vi "Untitled 3 (SubVI).vi"(8 "error in (no error)":errorcluster) -> (0 "error out":errorcluster, 2 "Array":u16[](array[numeric]), 3 "UP_Value":u16[](array[numeric]))   [LabVIEW 2016]
uses:
  <vilib>/myRIO/Instrument Drivers/Onboard IO/I2C/typedefs/I2C User Configuration.ctl
  <vilib>/myRIO/Instrument Drivers/Onboard IO/I2C/typedefs/I2C Transfer Rate.ctl
  <vilib>/myRIO/Instrument Drivers/Onboard IO/I2C/typedefs/I2C Reference.ctl
  <vilib>/myRIO/Common/Instrument Driver Framework/Utilities/typedefs/myRIO Generic Hardware Reference.ctl
  <vilib>/myRIO/Common/Instrument Driver Framework/Utilities/typedefs/Hardware Version Enum.ctl
  <vilib>/myRIO/Common/Instrument Driver Framework/Utilities/typedefs/myRIO v1.0 Reference.ctl
  <vilib>/myRIO/Common/Instrument Driver Framework/Utilities/typedefs/Generic FPGA Reference.ctl
  <vilib>/myRIO/Common/Instrument Driver Framework/myRIO v1.0/I2C/typedefs/I2C Channels Enum.ctl
  <vilib>/myRIO/Instrument Drivers/Onboard IO/I2C/typedefs/I2C Configuration.ctl
  <vilib>/userdefined/High Color/nirio_resource_hc.ctl
  <vilib>/myRIO/Common/Instrument Driver Framework/Utilities/vis/Is FPGA Ref Available.vi
  <vilib>/myRIO/Common/Instrument Driver Framework/myRIO v1.0/I2C/vis/myRIO v1.1 Open I2C.vi
  <vilib>/myRIO/Instrument Drivers/Onboard IO/I2C/vis/Configure.vi
  <vilib>/myRIO/Instrument Drivers/Onboard IO/I2C/vis/Write.vi
  <vilib>/myRIO/Instrument Drivers/Onboard IO/I2C/vis/Write Read.vi
  <vilib>/myRIO/Common/Instrument Driver Framework/Utilities/vis/Validate Channels.vi
  <vilib>/myRIO/Common/Instrument Driver Framework/myRIO v1.0/I2C/vis/myRIO v1.0 Reserve I2C.vi
  <vilib>/myRIO/Common/Instrument Driver Framework/myRIO v1.0/I2C/vis/myRIO v1.0 Build MUX Configuration I2C.vi
  <vilib>/myRIO/Common/Instrument Driver Framework/myRIO v1.0/Resource Manager/vis/myRIO v1.0 Reserve Channel List.vi
  <vilib>/myRIO/Common/Instrument Driver Framework/myRIO v1.0/Resource Manager/vis/myRIO v1.0 Create Configuration List.vi
  <vilib>/myRIO/Common/Instrument Driver Framework/myRIO v1.0/Resource Manager/vis/myRIO v1.0 Reserve Channel.vi
  <vilib>/myRIO/Common/Instrument Driver Framework/myRIO v1.0/Resource Manager/vis/myRIO v1.0 Unreserve Channel.vi
  <vilib>/myRIO/Common/Instrument Driver Framework/myRIO v1.0/Resource Manager/vis/myRIO v1.0 Build Mutex Name.vi
  <vilib>/Utility/VariantDataType/GetNumericInfo.vi
  <vilib>/Utility/error.llb/Error Cluster From Error Code.vi
  <vilib>/myRIO/Common/Instrument Driver Framework/myRIO v1.0/myRIO v1.1 Open.vi
  <vilib>/myRIO/Common/Instrument Driver Framework/Utilities/vis/IO Manager.vi
  <vilib>/myRIO/Common/Instrument Driver Framework/Utilities/vis/Configuration Manager.vi
  <vilib>/myRIO/Common/Instrument Driver Framework/myRIO v1.0/Resource Manager/vis/myRIO v1.0 Configure IO.vi
  <vilib>/myRIO/Common/Instrument Driver Framework/myRIO v1.0/myRIO v1.0 Close.vi
  <vilib>/myRIO/Common/Instrument Driver Framework/myRIO v1.0/I2C/vis/myRIO v1.0 Configure I2C.vi
  <vilib>/myRIO/Common/Instrument Driver Framework/myRIO v1.0/I2C/vis/myRIO v1.0 Write I2C.vi
  <vilib>/myRIO/Common/Instrument Driver Framework/myRIO v1.0/I2C/vis/myRIO v1.0 Read I2C.vi
  <vilib>/myRIO/Express VI/Onboard IO/I2C/I2C Express VI.xnode
  <vilib>/myRIO/Instrument Drivers/Onboard IO/I2C/vis/myRIO I2C Open.xnode
  <vilib>/myRIO/Instrument Drivers/Onboard IO/I2C/I2C.lvlib
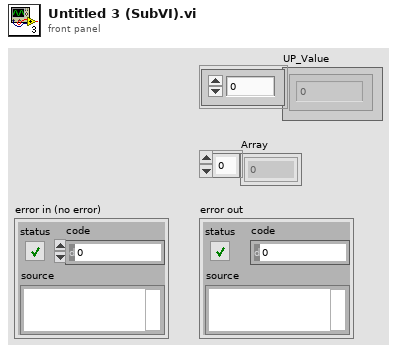
[diagram p1: front panel]
types:
  T1 = typedef "I2C.lvlib/I2C Reference.ctl" = cluster{"myRIO Reference":T2, "I2C Channels Enum":T6, "I2C Configuration":T7}
  T2 = typedef "myRIO Generic Hardware Reference.ctl" = cluster{"myRIO Model":T3, "myRIO Hardware Reference":T4}
  T3 = typedef "Hardware Version Enum.ctl" = enum16{"Unknown", "myRIO-1900", "myRIO-1950", "roboRIO", "NI ELVIS RIO CM"}
  T4 = typedef "myRIO v1.0 Reference.ctl" = cluster{"Generic FPGA Reference":T5, "Allow multiple opens":bool}
  T5 = typedef "Generic FPGA Reference.ctl" = refnum<k20>
  T6 = typedef "I2C Channels Enum.ctl" = enum16{"Not Connected", "A/I2C", "B/I2C", "I2C/I2C"}
  T7 = typedef "I2C.lvlib/I2C Configuration.ctl" = cluster{"I2C Transfer Rate":T8}
  T8 = typedef "I2C.lvlib/I2C Transfer Rate.ctl" = enum16{"Standard mode (100 kbps)", "Fast mode (400 kbps)"}
  T9 = typedef "I2C.lvlib/I2C User Configuration.ctl" = cluster{"I2C Transfer Rate":T8}
  T10 = typedef "nirio_resource_hc.ctl" = tag
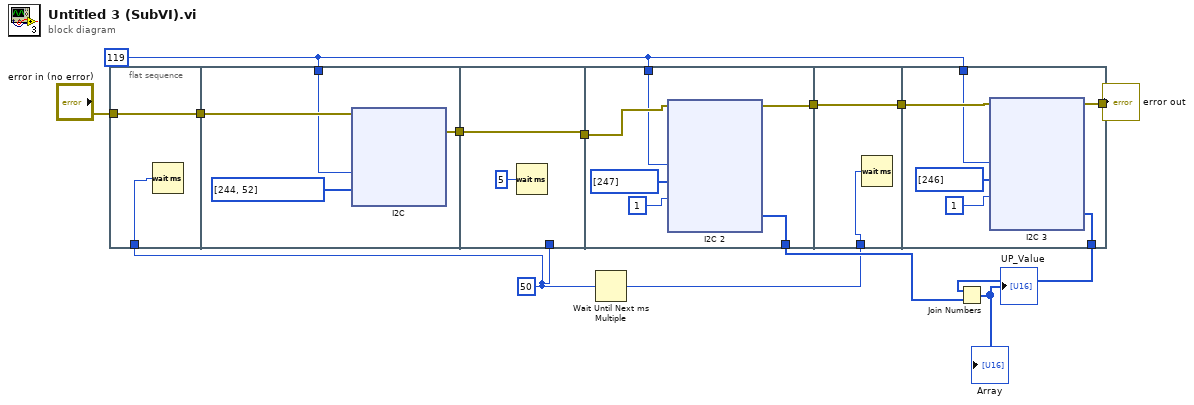
[diagram p0: block diagram]
diagram:
  w4 = u32 50 ("milliseconds to wait")
  w3 = u8 119 ("Slave Address (7-bit)")
  n1 = flat-sequence {
    tunnel: "error in (no error)" -> [w14]
    tunnel: [w14] -> w12
    tunnel: w4 -> [w13]
    tunnel: [w17] -> w11
    tunnel: w3 -> [w15]
    tunnel: w12 -> [w16]
    tunnel: [w58] -> w10
    tunnel: w11 -> [w58]
    tunnel: w4 -> [_]
    tunnel: w10 -> [w62]
    tunnel: [w61] -> w5
    tunnel: [w60] -> w9
    tunnel: w3 -> [w59]
    tunnel: w9 -> [w106]
    tunnel: [w106] -> w8
    tunnel: w4 -> [w105]
    tunnel: w8 -> [w110]
    tunnel: [w109] -> w2
    tunnel: w3 -> [w108]
    tunnel: [w107] -> w6
    frame #0 {
      n2 = Wait (ms)(milliseconds to wait=w13) -> ()  [unwired: 1 out]
    }
    frame #1 {
      n3 = xnode "I2C"("Slave Address (7-bit)"=w15, "Bytes to Write"=u8[] [244, 52], "error in (no error)"=w16) -> ("error out"=w17:errorcluster)
    }
    frame #2 {
      n4 = Wait (ms)(milliseconds to wait=u32 5 ("Zu wartende ms")) -> ()  [unwired: 1 out]
    }
    frame #3 {
      n5 = xnode "I2C 2"("Slave Address (7-bit)"=w59, "Bytes to Write"=u8[] [247], "Byte Count"=u8 1 ("Slave Address (7-bit)"), "error in (no error)"=w62) -> ("Bytes Read"=w61:u8[], "error out"=w60:errorcluster)
    }
    frame #4 {
      n6 = Wait (ms)(milliseconds to wait=w105) -> ()  [unwired: 1 out]
    }
    frame #5 {
      n7 = xnode "I2C 3"("Slave Address (7-bit)"=w108, "Bytes to Write"=u8[] [246], "Byte Count"=u8 1 ("Slave Address (7-bit)"), "error in (no error)"=w110) -> ("Bytes Read"=w107:u8[], "error out"=w109:errorcluster)
    }
  }
  n8 = Wait Until Next ms Multiple(millisecond multiple=w4) -> ()  [unwired: 1 out]
  n9 = Join Numbers(hi=w6, lo=w5) -> ((hi.lo)=→"UP_Value" →"Array":u16[])
  "error out" <- w2
